vi "ProtoGenerator.vi"(11 ".proto file path":path=path "C:/dev/labview-grpc-server/tests/data_marshal/data_marshal.proto") -> (1 "Messages":T1[](array[typedef]), 2 "Service Methods":T4(array[cluster]), 3 "Service Names":string[](array[string]))   [LabVIEW 2019]
uses:
  MessageMetadata.ctl
  MessageElementMetadata.ctl
  MessageElementType.ctl
  build/Debug/labview_grpc_generator.dll
  gprc-support.lvlib
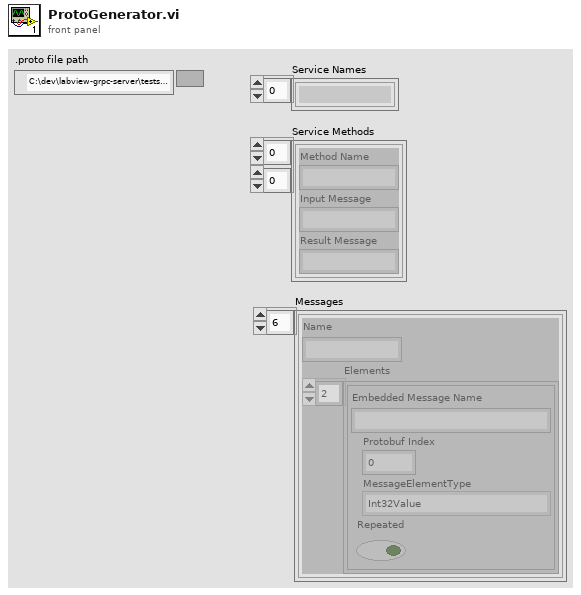
[diagram p1: front panel]
types:
  T1 = typedef "gprc-support.lvlib/MessageMetadata.ctl" = cluster{"Name":string, "Elements":T2[]}
  T2 = typedef "gprc-support.lvlib/MessageElementMetadata.ctl" = cluster{"Embedded Message Name":string, "Protobuf Index":i32, "MessageElementType":T3, "Repeated":bool}
  T3 = typedef "gprc-support.lvlib/MessageElementType.ctl" = enum32{"Int32Value", "FloatValue", "DoubleValue", "BoolValue", "StringValue", "MessageValue", ""}
  T4 = cluster{"Method Name":string, "Input Message":string, "Result Message":string}[][]
  T5 = cluster{"Method Name":string, "Input Message":string, "Result Message":string}
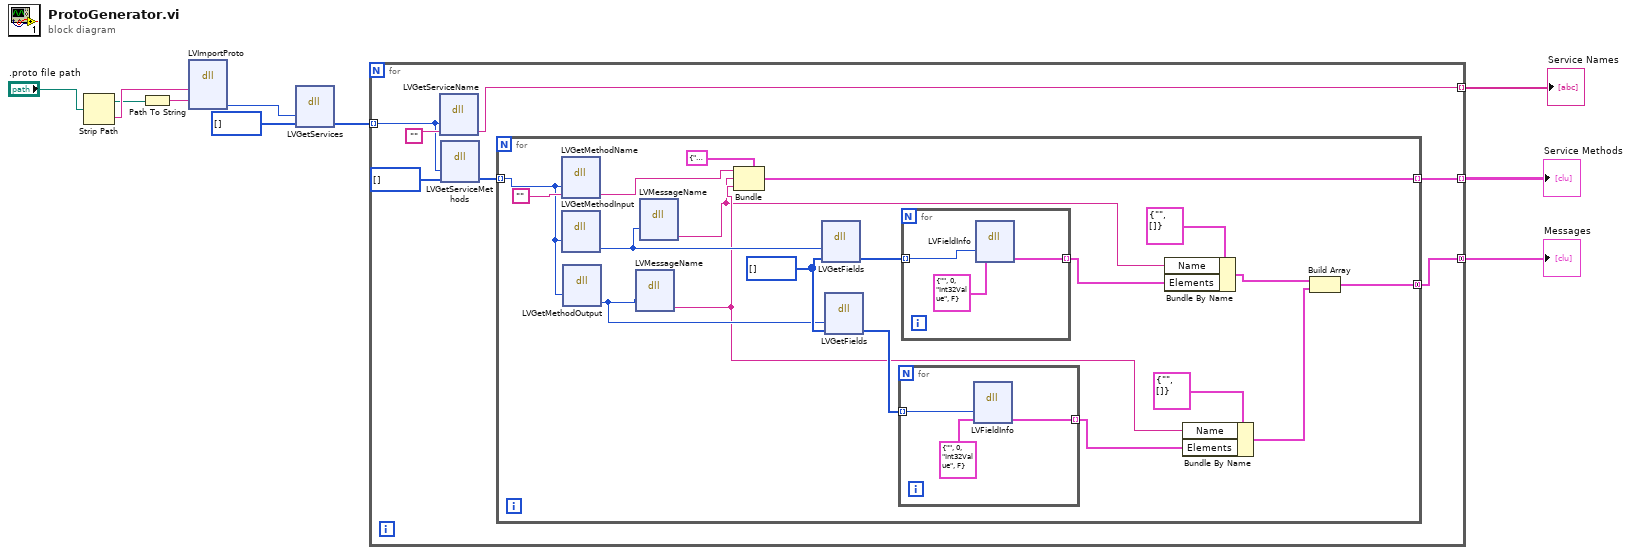
[diagram p0: block diagram]
diagram:
  n1 = Strip Path(path=".proto file path") -> (stripped path=w4:path, name=w5:string)
  n2 = Path To String(path=w4) -> (string=w3:string)
  n3 = dll-call lib="C:/dev/labview-grpc-server/build/Debug/labview_grpc_generator.dll" fn="LVImportProto"("protoName"=w5, "SearchPaths"=w3) -> ("protoDescription"=w9:u64)  [unwired: 7 in, 2 out]
  n4 = dll-call lib="C:/dev/labview-grpc-server/build/Debug/labview_grpc_generator.dll" fn="LVGetServices"("protoDescription"=w9, "services"=u64[] []) -> ("services"=w8:u64[])  [unwired: 5 in, 2 out]
  n5 = for {
    tunnel: w8 -> [w15] mode=indexing
    tunnel: [w13] -> w2 mode=indexing
    tunnel: [w12] -> w7 mode=indexing
    tunnel: [w11] -> w1 mode=concatenating
    n6 = dll-call lib="C:/dev/labview-grpc-server/build/Debug/labview_grpc_generator.dll" fn="LVGetServiceName"("service"=w15, "serviceName"="") -> ("serviceName"=w12:string)  [unwired: 5 in, 2 out]
    n7 = dll-call lib="C:/dev/labview-grpc-server/build/Debug/labview_grpc_generator.dll" fn="LVGetServiceMethods"("service"=w15, "serviceMethods"=u64[] []) -> ("serviceMethods"=w14:u64[])  [unwired: 5 in, 2 out]
    n8 = for {
      tunnel: w14 -> [w35] mode=indexing
      tunnel: [w28] -> w13 mode=indexing
      tunnel: [w18] -> w11 mode=concatenating
      w32 = u64[] []
      n9 = dll-call lib="C:/dev/labview-grpc-server/build/Debug/labview_grpc_generator.dll" fn="LVGetMethodName"("method"=w35, "methodName"="") -> ("methodName"=w29:string)  [unwired: 5 in, 2 out]
      n10 = dll-call lib="C:/dev/labview-grpc-server/build/Debug/labview_grpc_generator.dll" fn="LVGetMethodInput"("method"=w35) -> ("methodInput"=w27:u64)  [unwired: 6 in, 2 out]
      n11 = dll-call lib="C:/dev/labview-grpc-server/build/Debug/labview_grpc_generator.dll" fn="LVGetMethodOutput"("method"=w35) -> ("methodOutput"=w31:u64)  [unwired: 6 in, 2 out]
      n12 = dll-call lib="C:/dev/labview-grpc-server/build/Debug/labview_grpc_generator.dll" fn="LVMessageName"("message"=w31) -> ("name"=w24:string)  [unwired: 6 in, 2 out]
      n13 = dll-call lib="C:/dev/labview-grpc-server/build/Debug/labview_grpc_generator.dll" fn="LVMessageName"("message"=w27) -> ("name"=w22:string)  [unwired: 6 in, 2 out]
      n14 = Bundle(cluster=T5 {"Method Name"="", "Input Message"="", "Result Message"=""}, "Method Name"=w29, "Input Message"=w22, "Result Message"=w24) -> (w28:T5)
      n15 = dll-call lib="C:/dev/labview-grpc-server/build/Debug/labview_grpc_generator.dll" fn="LVGetFields"("message"=w27, "fieldInfo"=w32) -> ("fieldInfo"=w34:u64[])  [unwired: 5 in, 2 out]
      n16 = dll-call lib="C:/dev/labview-grpc-server/build/Debug/labview_grpc_generator.dll" fn="LVGetFields"("message"=w31, "fieldInfo"=w32) -> ("fieldInfo"=w33:u64[])  [unwired: 5 in, 2 out]
      n17 = for {
        tunnel: [w39] -> w25 mode=indexing
        tunnel: w33 -> [w38] mode=indexing
        n18 = dll-call lib="C:/dev/labview-grpc-server/build/Debug/labview_grpc_generator.dll" fn="LVFieldInfo"("field"=w38, T2 {"Embedded Message Name"="", "Protobuf Index"=0, "MessageElementType"=enum."Int32Value", "Repeated"=FALSE} ("MessageElementMetadata")) -> (w39:T2)  [unwired: 5 in, 2 out]
      }
      n19 = for {
        tunnel: w34 -> [w42] mode=indexing
        tunnel: [w41] -> w21 mode=indexing
        n20 = dll-call lib="C:/dev/labview-grpc-server/build/Debug/labview_grpc_generator.dll" fn="LVFieldInfo"("field"=w42, T2 {"Embedded Message Name"="", "Protobuf Index"=0, "MessageElementType"=enum."Int32Value", "Repeated"=FALSE} ("MessageElementMetadata")) -> (w41:T2)  [unwired: 5 in, 2 out]
      }
      n21 = Bundle By Name(cluster=T1 {"Name"="", "Elements"=[]} ("Message Metadata"), "Name"=w22, "Elements"=w21) -> (w20:T1)
      n22 = Bundle By Name(cluster=T1 {"Name"="", "Elements"=[]} ("Message Metadata"), "Name"=w24, "Elements"=w25) -> (w19:T1)
      n23 = Build Array(w20, w19) -> (w18:T1[])
    }
  }
  "Service Names" <- w7
  "Service Methods" <- w2
  "Messages" <- w1
